vi "Config dialog.vi"(8 "error in (no error)":errorcluster, 11 "DAQ module ID":i32) -> (0 "error out":errorcluster, 2 "Cancelled?":bool, 3 "DAQmx Device Name out":tag)   [LabVIEW 2020, in "UI.lvlib"]
uses:
  UI.lvlib
  Controls/Config diag states--typedef.ctl
  NI_DAQ/Libraries/NI DAQ/NI DAQ.lvlib
panel:
  in  "Cancel Button":bool
  in  "OK Button":bool
  out "Estado":string
  in  "Test Dev":bool
  in  "DAQ Device Name":tag
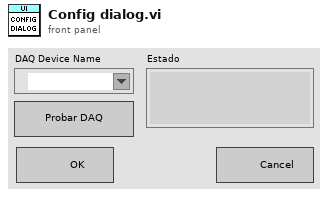
[diagram p1: front panel]
types:
  T1 = typedef "UI.lvlib/Config diag states--typedef.ctl" = enum16{"Initilialize", "Wait", "Exit"}
  T2 = enum8{"Enabled", "Disabled", "Disabled and Grayed Out"}
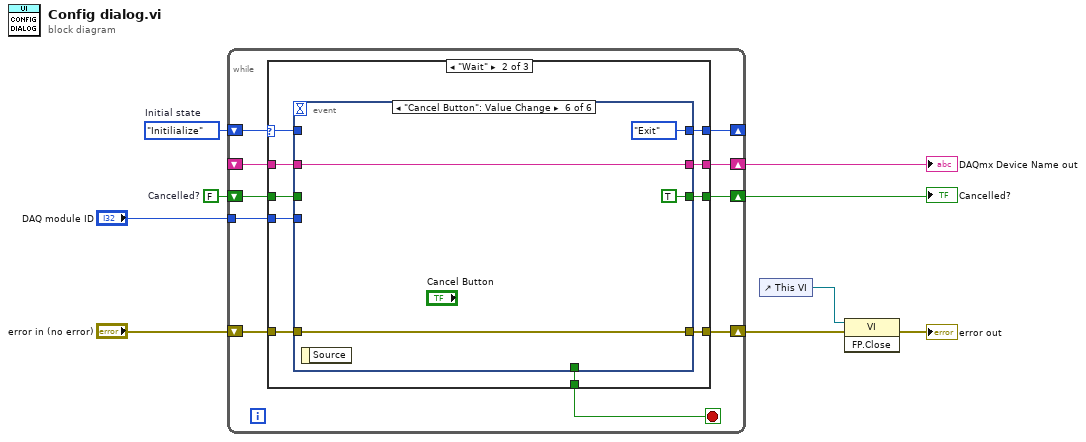
[diagram p0: block diagram]
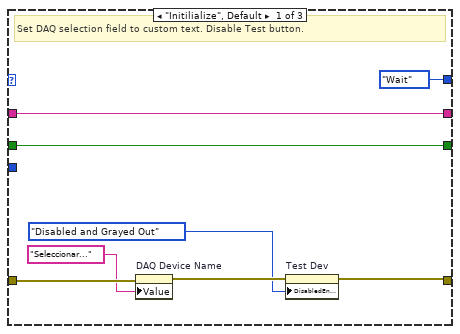
[diagram p2: hidden frame]
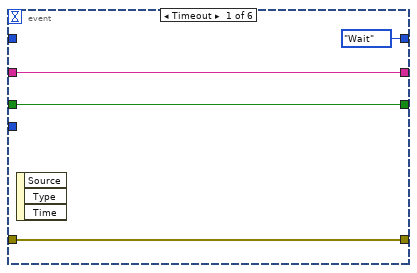
[diagram p3: hidden frame]
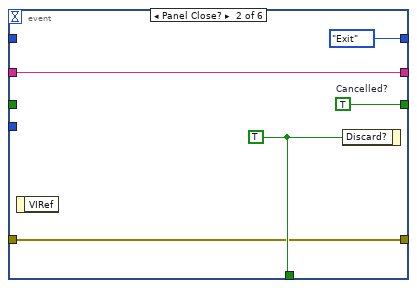
[diagram p4: hidden frame]
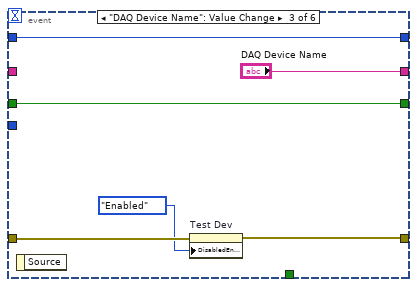
[diagram p5: hidden frame]
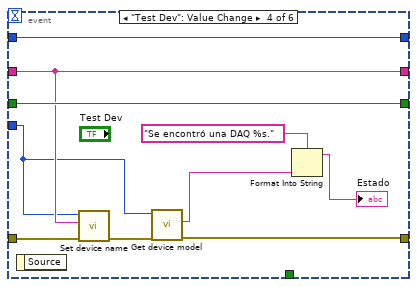
[diagram p6: hidden frame]
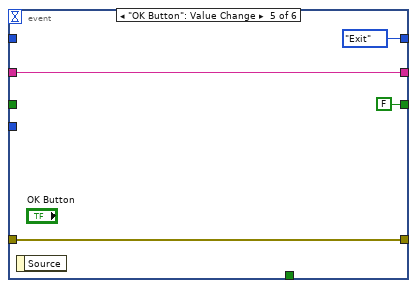
[diagram p7: hidden frame]
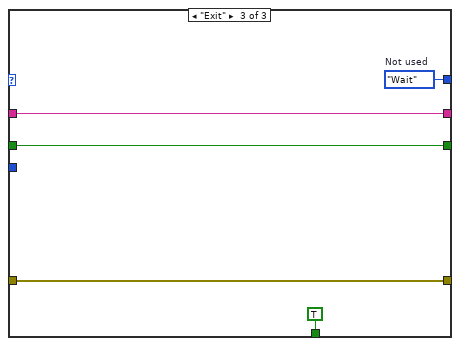
[diagram p8: hidden frame]
diagram:
  w7 = FALSE  # Cancelled?
  w9 = Config_diag_states--typedef."Initilialize"  # Initial state
  n1 = while {
    shift-right: [w17] -> w8
    shift-left: w7 -> [w16]
    shift-right: [w14] -> w3
    shift-left: "error in (no error)" -> [w15]
    shift-right: [w13] -> _
    shift-left: w9 -> [w19]
    tunnel: "DAQ module ID" -> [w12]
    shift-right: [w11] -> w4
    shift-left: _ -> [w10]
    stop <- w18 stop-if-true
    n2 = case shown="\"Wait\"" w19 {
      selector: w19 -> [_ w31 _]
      tunnel: [_ w37 TRUE ("Discard?")] -> w18
      tunnel: [w27 w36 w75] -> w17
      tunnel: w16 -> [w27 w35 w75]
      tunnel: w15 -> [w25 w34 w74]
      tunnel: [w21 w33 w74] -> w14
      tunnel: [Config_diag_states--typedef."Wait" w32 w72] -> w13
      tunnel: w12 -> [_ w28 _]
      tunnel: [w23 w30 w71] -> w11
      tunnel: w10 -> [w23 w29 w71]
      frame "Initilialize", Default {
        # "Set DAQ selection field to custom text. Disable Test button."
        n3 = property on="DAQ Device Name" class="DAQmxName"(error in=w25, "Value"="Seleccionar..." ("Value (Signaling)")) -> (error out=w22:errorcluster)  [unwired: 1 in, 1 out]
        n4 = property on="Test Dev" class="Bool"(error in=w22, "DisabledEnum"=T2."Disabled and Grayed Out" ("Disabled")) -> (error out=w21:errorcluster)  [unwired: 1 in, 1 out]
      }
      frame "Wait" {
        n5 = event shown="[5] \"Cancel Button\": Value Change" {
          selector: _ -> [_ _ _ _ _ _]
          dyn-events: _ -> [_ _ _ _ _ _]
          timeout: _ -> [_ _ _ _ _ _]
          tunnel: [_ w46 _ _ _ _] -> w37
          tunnel: [w41 w45 w52 w62 FALSE ("Cancelled?") TRUE ("Cancelled?")] -> w36
          tunnel: w35 -> [w41 _ w52 w62 _ _]
          tunnel: w34 -> [w40 w44 w49 w60 w66 w70]
          tunnel: [w40 w44 w48 w56 w66 w70] -> w33
          tunnel: [Config_diag_states--typedef."Wait" Config_diag_states--typedef."Exit" w51 w61 Config_diag_states--typedef."Exit" Config_diag_states--typedef."Exit"] -> w32
          tunnel: w31 -> [_ _ w51 w61 _ _]
          tunnel: [w38 w42 "DAQ Device Name" w59 w65 w69] -> w30
          tunnel: w29 -> [w38 w42 _ w59 w65 w69]
          tunnel: w28 -> [_ _ _ w57 _ _]
          event Timeout {
            n6 = event-data() -> ()  [unwired: 1 in, 3 out]
          }
          event Panel Close? {
            w45 = TRUE  # Cancelled?
            w46 = TRUE ("Discard?")
            n7 = event-data() -> ()  [unwired: 1 in, 1 out]
            n8 = event-data("Discard?"=w46) -> ()  [unwired: 1 in, 1 out]
          }
          event "DAQ Device Name": Value Change {
            n9 = event-data() -> ()  [unwired: 1 in, 1 out]
            n10 = property on="Test Dev" class="Bool"(error in=w49, "DisabledEnum"=T2."Enabled" ("Disabled")) -> (error out=w48:errorcluster)  [unwired: 1 in, 1 out]
          }
          event "Test Dev": Value Change {
            n11 = event-data() -> ()  [unwired: 1 in, 1 out]
            n12 = call "Set device name.vi"("error in"=w60, "Device name"=w59, "Module ID"=w57) -> ("error out"=w58:errorcluster)  [unwired: 8 in]
            n13 = call "Get device model.vi"("error in"=w58, "Module ID"=w57) -> ("error out"=w56:errorcluster, "Device model"=w54:string)  [unwired: 7 in, 1 out]
            n14 = Format Into String(format string="Se encontró una DAQ %s.", w54) -> (resulting string=→"Estado":string)  [unwired: 2 in, 1 out]
          }
          event "OK Button": Value Change {
            n15 = event-data() -> ()  [unwired: 1 in, 1 out]
          }
          event "Cancel Button": Value Change {
            n16 = event-data() -> ()  [unwired: 1 in, 1 out]
          }
        }
      }
      frame "Exit" {
        w72 = Config_diag_states--typedef."Wait"  # Not used
      }
    }
  }
  "Cancelled?" <- w8
  "DAQmx Device Name out" <- w4
  n17 = control-ref of="This VI"() -> (w1:refnum<vi>)
  n18 = invoke class="VI" method="FP.Close"(reference=w1, error in=w3) -> (error out=→"error out":errorcluster)  [unwired: 1 in, 2 out]
